vi "ImportSession.vi"(4 "notes":string, 5 "file_name":string, 6 "depth":dbl, 7 "pulse_duration":dbl, 8 "error in (no error)":errorcluster, 9 "mouse_id":dbl, 10 "intertrial_interval":dbl, 11 "Acquisition in":refnum<class "Acquisition.lvclass">) -> (0 "error out":errorcluster, 3 "Acquisition out":refnum<class "Acquisition.lvclass">)   [LabVIEW 2014, in "Acquisition.lvclass"]
uses:
  Acquisition.lvclass
  Acquisition.lvclass/Acquisition.ctl
  Database/Database.lvclass
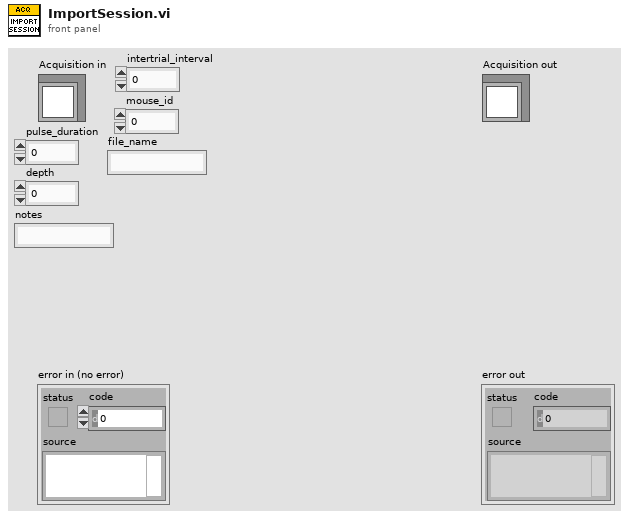
[diagram p1: front panel]
types:
  T1 = cluster{"mouse_id":dbl, "session_timestamp":string, "pulse_duration":dbl, "intertrial_interval":dbl, "file_name":string, "depth":dbl, "notes":string}
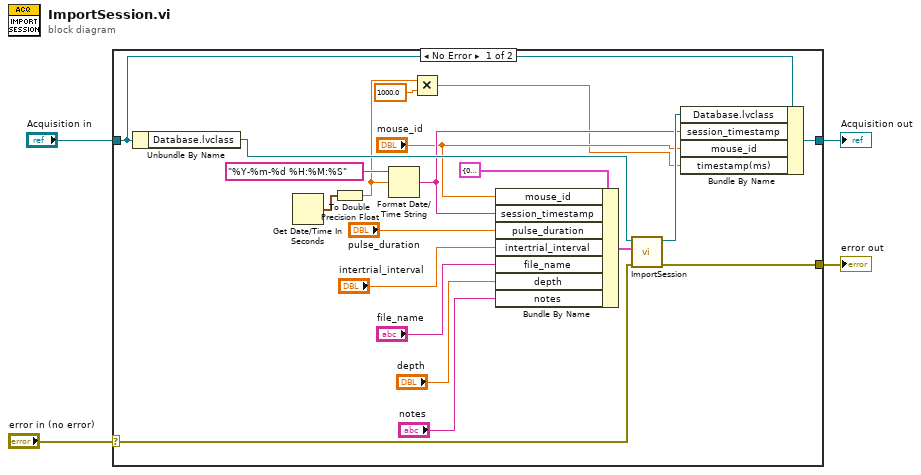
[diagram p0: block diagram]
diagram:
  n1 = case shown="No Error" "error in (no error)" {
    selector: "error in (no error)" -> [w18 w26]
    tunnel: [w14 w26] -> w3
    tunnel: [w16 w25] -> w1
    tunnel: "Acquisition in" -> [w17 w25]
    frame No Error {
      n2 = Unbundle By Name(w17) -> ("Database.lvclass"=w22:refnum<class "Database.lvclass">)
      n3 = Get Date/Time In Seconds() -> (seconds since 1Jan1904=w23:timestamp)
      n4 = To Double Precision Float(number=w23) -> (double precision float=w5:dbl)
      n5 = Format Date/Time String(time format string (%c)="%Y-%m-%d %H:%M:%S", seconds (now)=w5) -> (date/time string=w13:string)  [unwired: 1 in]
      n6 = Multiply(x=w5, y=1000.0) -> (x*y=w6:dbl)
      n7 = Bundle By Name(cluster=T1 {"mouse_id"=0.0, "session_timestamp"="2016-04-18 12:39:42", "pulse_duration"=4000.0, "intertrial_interval"=4000.0, "file_name"="", "depth"=0.0, "notes"=""} ("Tuple"), "mouse_id"="mouse_id", "session_timestamp"=w13, "pulse_duration"="pulse_duration", "intertrial_interval"="intertrial_interval", "file_name"="file_name", "depth"="depth", "notes"="notes") -> (w19:T1)
      n8 = call-dynamic "ImportSession.vi"("error in (no error)"=w18, "Tuple"=w19, "Database in"=w22) -> ("error out"=w14:errorcluster, "Database out"=w15:refnum<class "Database.lvclass">)  [unwired: 7 in]
      n9 = Bundle By Name(cluster=w17, "Database.lvclass"=w15, "session_timestamp"=w13, "mouse_id"="mouse_id", "timestamp(ms)"=w6) -> (w16:refnum<class "Acquisition.lvclass">)
    }
    frame Error {
    }
  }
  "error out" <- w3
  "Acquisition out" <- w1
